vi "Solve Complex Linear Eqs (Gen, single right hand).vi"(9 "relative tolerance":dbl=-1.0, 10 "Known Vector":cdb[](array[numeric]), 11 "Input Matrix":T1) -> (0 "error":i32, 3 "Solution Vector":cdb[](array[numeric]))   [LabVIEW 2020, in "NI_AALPro.lvlib"]
uses:
  <vilib>/Analysis/NI_AALPro.lvlib
  <vilib>/Analysis/Matrix/Datatypes/ComplexMatrix.ctl
  <vilib>/Analysis/NI_AALBase.lvlib
  <vilib>/Analysis/Matrix/NI_Matrix.lvlib
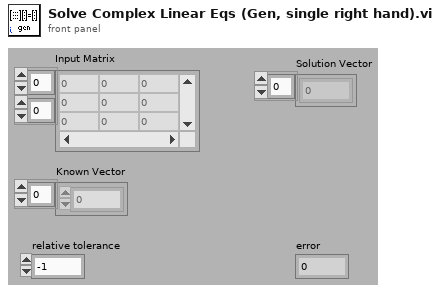
[diagram p1: front panel]
types:
  T1 = typedef "NI_Matrix.lvlib/ComplexMatrix.ctl" = cdb[][]
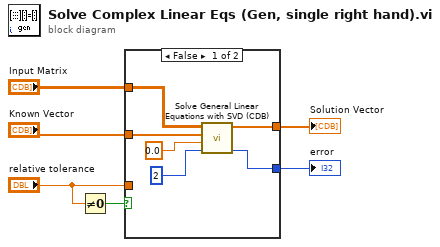
[diagram p0: block diagram]
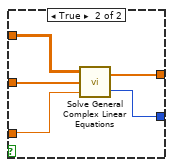
[diagram p2: hidden frame]
diagram:
  n1 = Not Equal To 0?(x="relative tolerance") -> (x != 0?=w6:bool)
  n2 = case shown="False" w6 {
    tunnel: "relative tolerance" -> [_ w15]
    tunnel: "Known Vector" -> [w11 w16]
    tunnel: "Input Matrix" -> [w12 w17]
    tunnel: [w7 w13] -> w2
    tunnel: [w8 w14] -> w1
    frame False {
      n3 = call <vilib>:"Solve General Linear Equations with SVD (CDB).vi"("iteration"=2, "relative tolerance"=0.0, "Known Vector"=w11, "Input Matrix"=w12) -> ("error"=w7:i32, "Solution Vector"=w8:cdb[])  [unwired: 6 in]
    }
    frame True {
      n4 = call <vilib>:"Solve General Complex Linear Equations.vi"("relative tolerance"=w15, "Known Vector"=w16, "Input Matrix"=w17) -> ("error"=w13:i32, "Solution Vector"=w14:cdb[])
    }
  }
  "Solution Vector" <- w1
  "error" <- w2
